vi "getRegisters.vi"(0 "AddressSpace":refnum<class "AddressSpace.lvclass">) -> (4 "registers":T1={"PLLGains"="PLLGains", "PLLRange"="PLLRange", "PLL_reset"="PLL_reset", "PLL_locked"="PLL_locked", "freqBoundaries"="freqBoundaries", "expectedFreq"="expectedFreq", "lockDuration"="lockDuration", "dT"="dT", "detectedFreq"="detectedFreq", "adjustTheta"="adjustTheta", "HarmonicFilter"="HarmonicFilter", "HarmonicFilterEnable"="HarmonicFilterEnable"})   [LabVIEW 2017, in "ThreePhasePLL.lvlib" / "AddressSpace.lvclass"]
uses:
  AddressSpace.lvclass
  registers.ctl
  AddressSpace.lvclass/AddressSpace.ctl
  ThreePhasePLL.lvlib
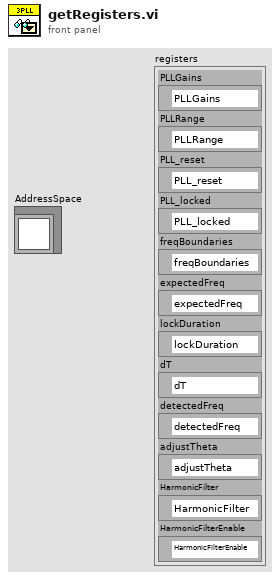
[diagram p1: front panel]
types:
  T1 = typedef "ThreePhasePLL.lvlib/registers.ctl" = cluster{"PLLGains":refnum<k21>, "PLLRange":refnum<k21>, "PLL_reset":refnum<k21>, "PLL_locked":refnum<k21>, "freqBoundaries":refnum<k21>, "expectedFreq":refnum<k21>, "lockDuration":refnum<k21>, "dT":refnum<k21>, "detectedFreq":refnum<k21>, "adjustTheta":refnum<k21>, "HarmonicFilter":refnum<k21>, "HarmonicFilterEnable":refnum<k21>}
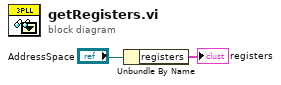
[diagram p0: block diagram]
diagram:
  n1 = Unbundle By Name("AddressSpace") -> ("registers"=→"registers":T1)
